vi "ArmCurls.vi"() -> ()   [LabVIEW 2018]
panel:
  in  "ShoulderSpeed":dbl
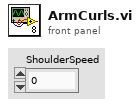
[diagram p1: front panel]
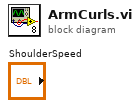
[diagram p0: block diagram]
diagram:
